vi "MeasLeakRate10.vi"() -> ()   [LabVIEW 2011]
panel:
  out "T-T0,P":cluster{"element":dbl, "element":dbl}[](array[cluster])
  out "t0":dbl format="%#_8f"
  out "XY Graph":cluster{"element":dbl, "element":dbl}[](graph)
  out "S00":i32
  out "S20":dbl
  out "S11":dbl
  out "S10":dbl
  out "S01":dbl
  out "T,P":cluster{"element":dbl, "element":dbl}[](array[cluster])
  out "dPdt":dbl
  out "Pavg":dbl
  out "average P (Torr)":string
  in  "Control Valve local":bool
  in  "Exhaust Local":bool
  in  "Exhaust Close":bool
  in  "Exhaust Open":bool
  in  "Control Close":bool
  in  "Control Open":bool
  in  "reset":bool
  in  "# points to watch":i32=60
  out "leak rate (Torr/min)":string
  out "P":dbl
  out "first":bool=TRUE
  in  "interval (s)":dbl=0.5
  in  "stop":bool
  out "P(Torr)":string
  # "Pressure control valve:"
  # "Exahaust valve:"
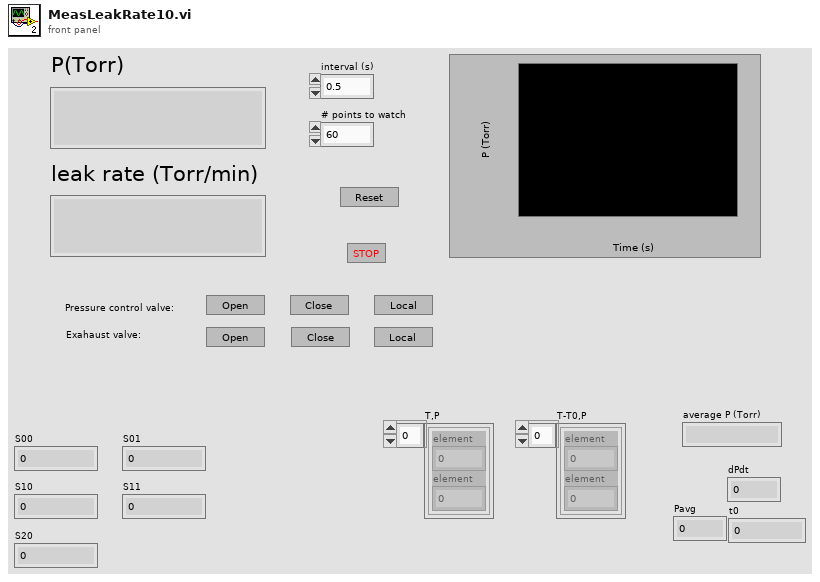
[diagram p1: front panel]
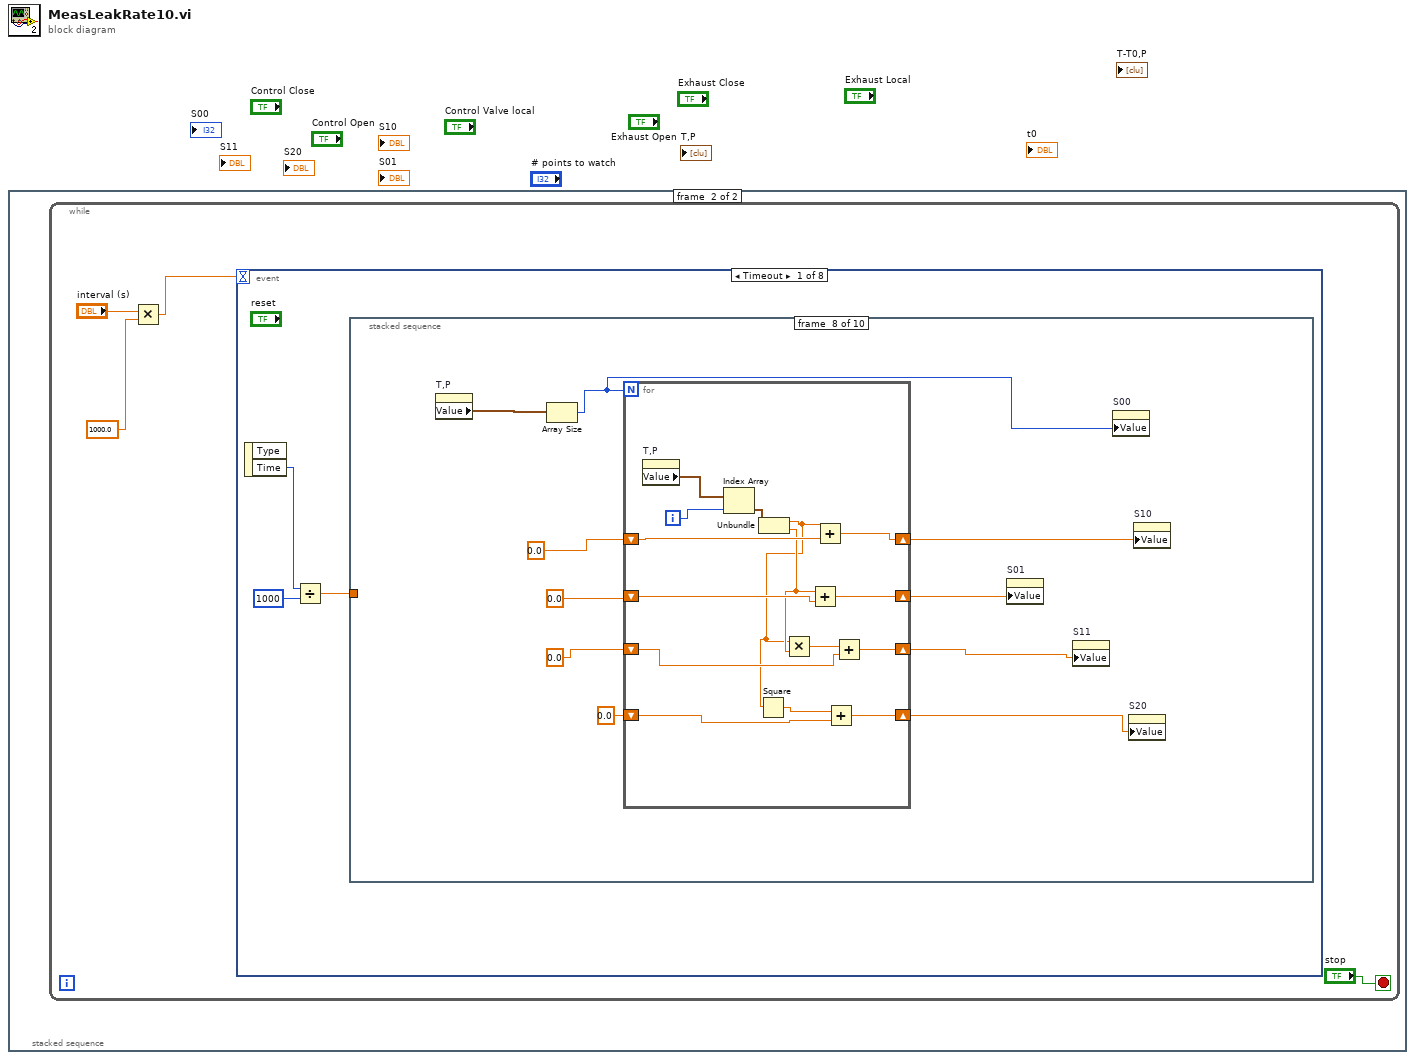
[diagram p0: block diagram]
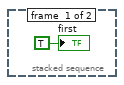
[diagram p2: hidden frame]
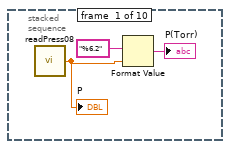
[diagram p3: hidden frame]
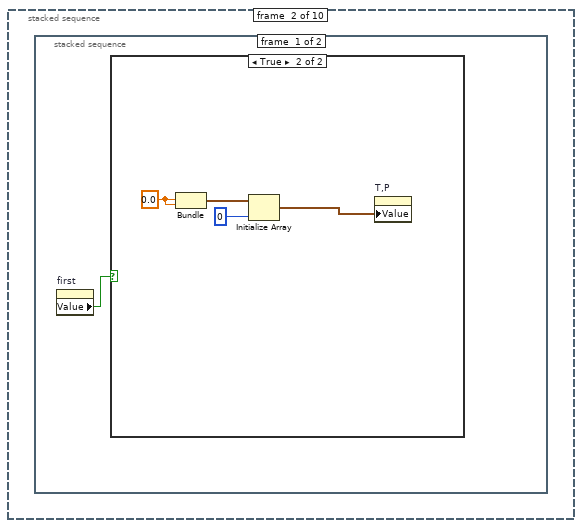
[diagram p4: hidden frame]
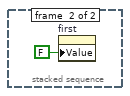
[diagram p6: hidden frame]
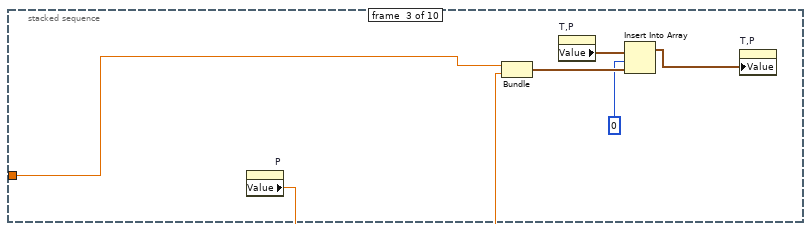
[diagram p7: hidden frame]
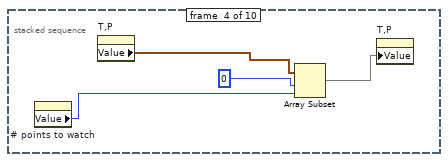
[diagram p8: hidden frame]
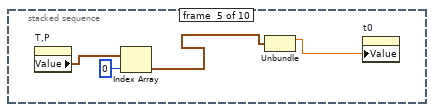
[diagram p9: hidden frame]
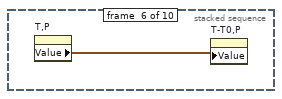
[diagram p10: hidden frame]
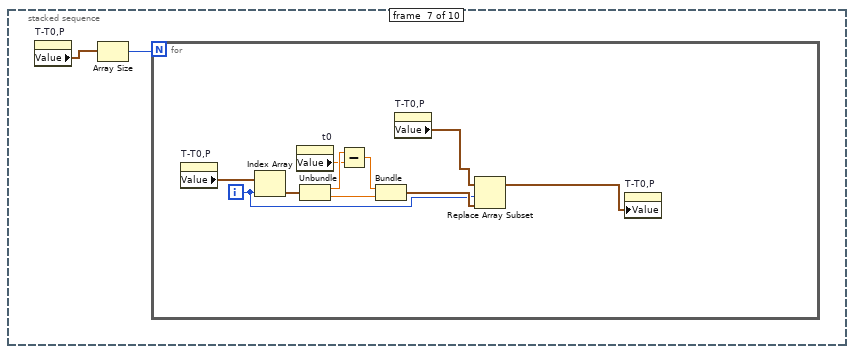
[diagram p11: hidden frame]
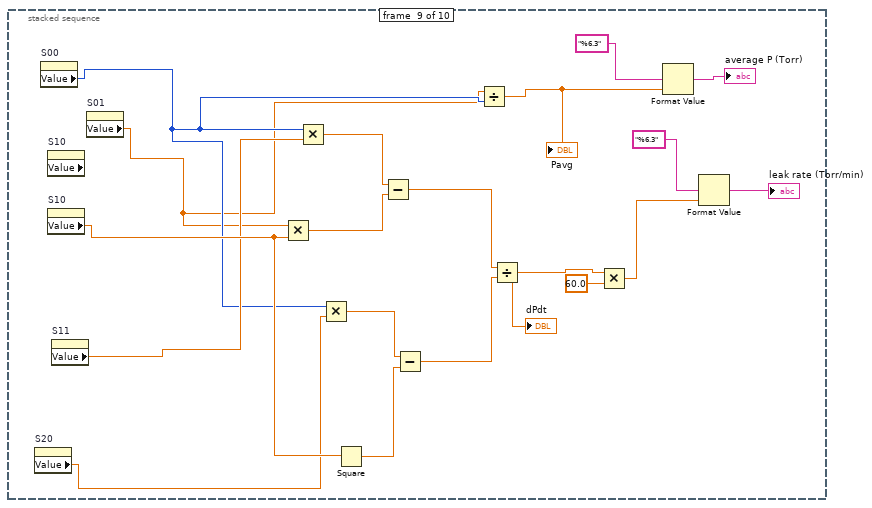
[diagram p12: hidden frame]
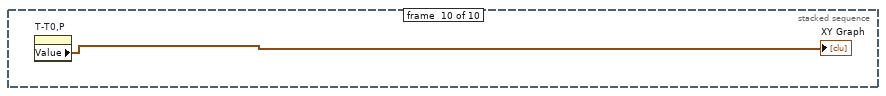
[diagram p13: hidden frame]
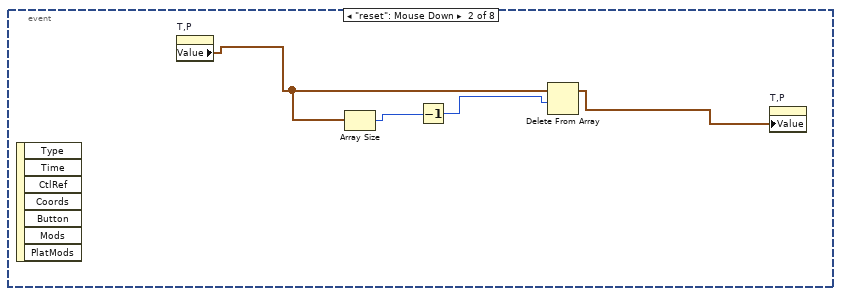
[diagram p14: hidden frame]
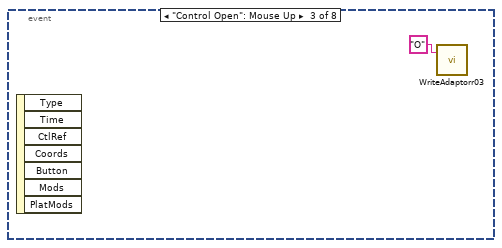
[diagram p15: hidden frame]
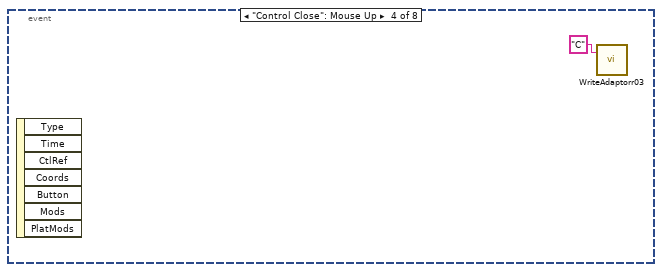
[diagram p16: hidden frame]
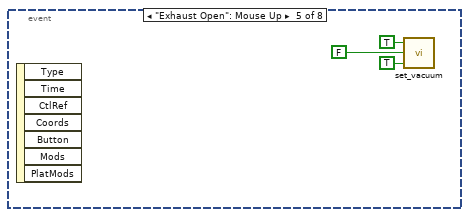
[diagram p17: hidden frame]
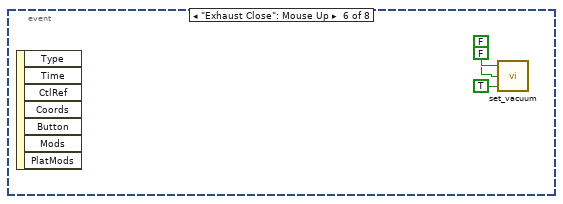
[diagram p18: hidden frame]
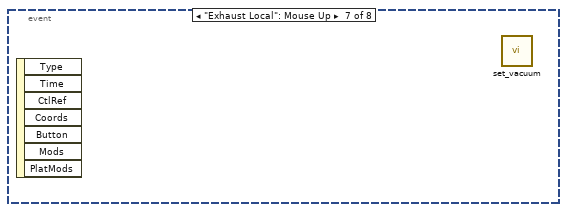
[diagram p19: hidden frame]
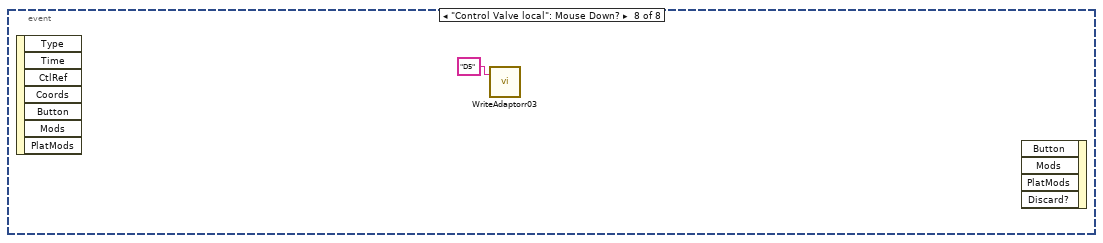
[diagram p20: hidden frame]
diagram:
  n1 = stacked-sequence {
    frame #0 {
      "first" <- TRUE ("first")
    }
    frame #1 {
      n2 = while {
        stop <- "stop" stop-if-true
        n3 = Multiply(x="interval (s)", y=1000.0) -> (x*y=w3:dbl)
        n4 = event shown="[0] Timeout" {
          selector: _ -> [_ _ _ _ _ _ _ _]
          dyn-events: _ -> [_ _ _ _ _ _ _ _]
          timeout: w3 -> [_ _ _ _ _ _ _ _]
          event Timeout {
            n5 = event-data() -> ("Time"=w8:u32)  [unwired: 1 in, 1 out]
            n6 = Divide(x=w8, y=u32 1000) -> (x/y=w6:dbl)
            n7 = stacked-sequence {
              tunnel: w6 -> [_ _ w23 _ _ _ _ _ _ _]
              frame #0 {
                n8 = call "readPress08.vi"() -> ("P"=w10:dbl)
                "P" <- w10
                n9 = Format Value(format string="%6.2", value (0)=w10) -> (output string=→"P(Torr)":string)  [unwired: 1 in]
              }
              frame #1 {
                n10 = stacked-sequence {
                  frame #0 {
                    n11 = property on="first" class="Bool (strict)"() -> ("Value"=w12:bool)  [unwired: 2 in, 2 out]
                    n12 = case shown="True" w12 {
                      frame False {
                      }
                      frame True {
                        w15 = 0.0 ("element")
                        n13 = Bundle("element"=w15, "element"=w15) -> (w14:cluster{"element":dbl, "element":dbl})  [unwired: 1 in]
                        n14 = Initialize Array(w14, 0 ("dimension size")) -> (w13:cluster{"element":dbl, "element":dbl}[])
                        n15 = property on="T,P" class="Arr (strict)"("Value"=w13) -> ()  [unwired: 2 in, 2 out]
                      }
                    }
                  }
                  frame #1 {
                    n16 = property on="first" class="Bool (strict)"("Value"=FALSE ("first")) -> ()  [unwired: 2 in, 2 out]
                  }
                }
              }
              frame #2 {
                n17 = property on="P" class="DigNum (strict)"() -> ("Value"=w22:dbl)  [unwired: 2 in, 2 out]
                n18 = Bundle(w23, "Value"=w22) -> (w20:cluster{dbl, "Value":dbl})  [unwired: 1 in]
                n19 = property on="T,P" class="Arr (strict)"() -> ("Value"=w21:cluster{"element":dbl, "element":dbl}[])  [unwired: 2 in, 2 out]
                n20 = Insert Into Array(array=w21, index=0, new element=w20) -> (w18:cluster{"element":dbl, "element":dbl}[])
                n21 = property on="T,P" class="Arr (strict)"("Value"=w18) -> ()  [unwired: 2 in, 2 out]
              }
              frame #3 {
                n22 = property on="# points to watch" class="DigNum (strict)"() -> ("Value"=w25:i32)  [unwired: 2 in, 2 out]
                n23 = property on="T,P" class="Arr (strict)"() -> ("Value"=w26:cluster{"element":dbl, "element":dbl}[])  [unwired: 2 in, 2 out]
                n24 = Array Subset(array=w26, index=0, length=w25) -> (w24:cluster{"element":dbl, "element":dbl}[])
                n25 = property on="T,P" class="Arr (strict)"("Value"=w24) -> ()  [unwired: 2 in, 2 out]
              }
              frame #4 {
                n26 = property on="T,P" class="Arr (strict)"() -> ("Value"=w31:cluster{"element":dbl, "element":dbl}[])  [unwired: 2 in, 2 out]
                n27 = Index Array(array=w31, index=0) -> (element=w29:cluster{"element":dbl, "element":dbl})
                n28 = Unbundle(w29) -> ("element"=w28:dbl)  [unwired: 1 out]
                n29 = property on="t0" class="DigNum (strict)"("Value"=w28) -> ()  [unwired: 2 in, 2 out]
              }
              frame #5 {
                n30 = property on="T,P" class="Arr (strict)"() -> ("Value"=w32:cluster{"element":dbl, "element":dbl}[])  [unwired: 2 in, 2 out]
                n31 = property on="T-T0,P" class="Arr (strict)"("Value"=w32) -> ()  [unwired: 2 in, 2 out]
              }
              frame #6 {
                n32 = property on="T-T0,P" class="Arr (strict)"() -> ("Value"=w34:cluster{"element":dbl, "element":dbl}[])  [unwired: 2 in, 2 out]
                n33 = Array Size(array=w34) -> (size(s)=w33:i32)
                n34 = for {
                  N: w33 -> [_]
                  i -> [w35]
                  n35 = property on="T-T0,P" class="Arr (strict)"() -> ("Value"=w39:cluster{"element":dbl, "element":dbl}[])  [unwired: 2 in, 2 out]
                  n36 = Index Array(array=w39, index=w35) -> (element=w44:cluster{"element":dbl, "element":dbl})
                  n37 = property on="t0" class="DigNum (strict)"() -> ("Value"=w42:dbl)  [unwired: 2 in, 2 out]
                  n38 = Unbundle(w44) -> ("element"=w43:dbl, "element"=w40:dbl)
                  n39 = Subtract(x=w43, y=w42) -> (x-y=w41:dbl)
                  n40 = Bundle(w41, "element"=w40) -> (w38:cluster{dbl, "element":dbl})  [unwired: 1 in]
                  n41 = property on="T-T0,P" class="Arr (strict)"() -> ("Value"=w37:cluster{"element":dbl, "element":dbl}[])  [unwired: 2 in, 2 out]
                  n42 = Replace Array Subset(array=w37, new element=w38, index=w35) -> (w36:cluster{"element":dbl, "element":dbl}[])
                  n43 = property on="T-T0,P" class="Arr (strict)"("Value"=w36) -> ()  [unwired: 2 in, 2 out]
                }
              }
              frame #7 {
                n44 = property on="T,P" class="Arr (strict)"() -> ("Value"=w53:cluster{"element":dbl, "element":dbl}[])  [unwired: 2 in, 2 out]
                n45 = Array Size(array=w53) -> (size(s)=w48:i32)
                n46 = for {
                  N: w48 -> [_]
                  shift-right: [w67] -> w47
                  shift-left: 0.0 -> [w69]
                  shift-right: [w65] -> w51
                  shift-left: 0.0 -> [w64]
                  shift-right: [w61] -> w46
                  shift-left: 0.0 -> [w60]
                  shift-right: [w57] -> w45
                  shift-left: 0.0 -> [w56]
                  i -> [w55]
                  n47 = property on="T,P" class="Arr (strict)"() -> ("Value"=w66:cluster{"element":dbl, "element":dbl}[])  [unwired: 2 in, 2 out]
                  n48 = Index Array(array=w66, index=w55) -> (element=w68:cluster{"element":dbl, "element":dbl})
                  n49 = Unbundle(w68) -> ("element"=w59:dbl, "element"=w63:dbl)
                  n50 = Square(x=w59) -> (x^2=w58:dbl)
                  n51 = Multiply(x=w59, y=w63) -> (x*y=w62:dbl)
                  n52 = Add(x=w63, y=w64) -> (x+y=w65:dbl)
                  n53 = Add(x=w59, y=w69) -> (x+y=w67:dbl)
                  n54 = Add(x=w58, y=w56) -> (x+y=w57:dbl)
                  n55 = Add(x=w62, y=w60) -> (x+y=w61:dbl)
                }
                n56 = property on="S01" class="DigNum (strict)"("Value"=w51) -> ()  [unwired: 2 in, 2 out]
                n57 = property on="S11" class="DigNum (strict)"("Value"=w46) -> ()  [unwired: 2 in, 2 out]
                n58 = property on="S00" class="DigNum (strict)"("Value"=w48) -> ()  [unwired: 2 in, 2 out]
                n59 = property on="S20" class="DigNum (strict)"("Value"=w45) -> ()  [unwired: 2 in, 2 out]
                n60 = property on="S10" class="DigNum (strict)"("Value"=w47) -> ()  [unwired: 2 in, 2 out]
              }
              frame #8 {
                n61 = property on="S20" class="DigNum (strict)"() -> ("Value"=w72:dbl)  [unwired: 2 in, 2 out]
                n62 = property on="S00" class="DigNum (strict)"() -> ("Value"=w71:i32)  [unwired: 2 in, 2 out]
                n63 = property on="S10" class="DigNum (strict)" props=["Value"]() -> ()  [unwired: 2 in, 3 out]
                n64 = property on="S10" class="DigNum (strict)"() -> ("Value"=w74:dbl)  [unwired: 2 in, 2 out]
                n65 = property on="S11" class="DigNum (strict)"() -> ("Value"=w73:dbl)  [unwired: 2 in, 2 out]
                n66 = property on="S01" class="DigNum (strict)"() -> ("Value"=w70:dbl)  [unwired: 2 in, 2 out]
                n67 = Multiply(x=w70, y=w74) -> (x*y=w87:dbl)
                n68 = Multiply(x=w71, y=w73) -> (x*y=w88:dbl)
                n69 = Multiply(x=w71, y=w72) -> (x*y=w86:dbl)
                n70 = Square(x=w74) -> (x^2=w85:dbl)
                n71 = Subtract(x=w88, y=w87) -> (x-y=w84:dbl)
                n72 = Subtract(x=w86, y=w85) -> (x-y=w83:dbl)
                n73 = Divide(x=w70, y=w71) -> (x/y=w77:dbl)
                "Pavg" <- w77
                n74 = Divide(x=w84, y=w83) -> (x/y=w82:dbl)
                "dPdt" <- w82
                n75 = Multiply(x=w82, y=60.0) -> (x*y=w78:dbl)
                n76 = Format Value(format string="%6.3", value (0)=w77) -> (output string=→"average P (Torr)":string)  [unwired: 1 in]
                n77 = Format Value(format string="%6.3", value (0)=w78) -> (output string=→"leak rate (Torr/min)":string)  [unwired: 1 in]
              }
              frame #9 {
                n78 = property on="T-T0,P" class="Arr (strict)"() -> ("Value"=→"XY Graph":cluster{"element":dbl, "element":dbl}[])  [unwired: 2 in, 2 out]
              }
            }
          }
          event "reset": Mouse Down {
            n79 = event-data() -> ()  [unwired: 1 in, 7 out]
            n80 = property on="T,P" class="Arr (strict)"() -> ("Value"=w91:cluster{"element":dbl, "element":dbl}[])  [unwired: 2 in, 2 out]
            n81 = Array Size(array=w91) -> (size(s)=w93:i32)
            n82 = Decrement(x=w93) -> (x-1=w92:i32)
            n83 = Delete From Array(array=w91, length=w92) -> (array with subset deleted=w90:cluster{"element":dbl, "element":dbl}[])  [unwired: 1 in, 1 out]
            n84 = property on="T,P" class="Arr (strict)"("Value"=w90) -> ()  [unwired: 2 in, 2 out]
          }
          event "Control Open": Mouse Up {
            n85 = event-data() -> ()  [unwired: 1 in, 7 out]
            n86 = call "WriteAdaptorr03.vi"("string to write"="O") -> ()  [unwired: 1 in, 1 out]
          }
          event "Control Close": Mouse Up {
            n87 = event-data() -> ()  [unwired: 1 in, 7 out]
            n88 = call "WriteAdaptorr03.vi"("string to write"="C") -> ()  [unwired: 1 in, 1 out]
          }
          event "Exhaust Open": Mouse Up {
            n89 = event-data() -> ()  [unwired: 1 in, 7 out]
            n90 = call "set_vacuum.vi"("Vac Remote"=TRUE, "Atm Exhaust"=FALSE, "Vac Exhaust"=TRUE) -> ()
          }
          event "Exhaust Close": Mouse Up {
            n91 = event-data() -> ()  [unwired: 1 in, 7 out]
            n92 = call "set_vacuum.vi"("Vac Remote"=TRUE, "Atm Exhaust"=FALSE, "Vac Exhaust"=FALSE) -> ()
          }
          event "Exhaust Local": Mouse Up {
            n93 = event-data() -> ()  [unwired: 1 in, 7 out]
            n94 = call "set_vacuum.vi"() -> ()  [unwired: 3 in]
          }
          event "Control Valve local": Mouse Down? {
            n95 = event-data() -> ()  [unwired: 1 in, 7 out]
            n96 = call "WriteAdaptorr03.vi"("string to write"="D5") -> ()  [unwired: 1 in, 1 out]
            n97 = event-data() -> ()  [unwired: 5 in, 1 out]
          }
        }
      }
    }
  }
